vi "20150905 gyro+accel+ UL sensor+servo test.vi"() -> ()   [LabVIEW 2013]
uses:
  <vilib>/MakerHub/LINX/Public/Sensors/Accelerometer/MPU60X0/DeviceAddresses.ctl
  <vilib>/Analysis/baseanly.llb/Mean (DBL).vi
  <vilib>/MakerHub/LINX/Public/Sensors/Motion/Servo/Servo Open N Channels.vi
  <vilib>/MakerHub/LINX/Public/Sensors/Motion/Servo/Servo Close N Channels.vi
  <vilib>/MakerHub/LINX/Public/Sensors/Motion/Servo/Servo Set Pulse Width N Channels.vi
  <vilib>/addons/Time Series Analysis/Series Preprocess.llb/TSA Moving Average (Array).vi
  <vilib>/MakerHub/LINX/LMH-LINX.lvlib
  <vilib>/MakerHub/LINX/Public/Sensors/Motion/Servo/Servo.lvlib
  <vilib>/MakerHub/LINX/Public/Sensors/Ultrasonic/Ultrasonic.lvlib
  <vilib>/MakerHub/LINX/Public/Sensors/Accelerometer/MPU60X0/MPU60X0.lvlib
  <vilib>/addons/_Advanced Signal Processing/NI_AdvSigProcTSA.lvlib
  <vilib>/Analysis/NI_AALBase.lvlib
panel:
  in  "Moving avg?":bool
  out "Error Out":errorcluster
  out "Waveform Chart":cluster{"mean":dbl, "mean":dbl, "mean":dbl}(graph)
  out "mean 3":dbl format="%0.2f"
  out "mean 2":dbl format="%0.2f"
  out "mean":dbl format="%0.2f"
  out "x/y":T1
  in  "Servo Channels":u8[](array[numeric])=[2, 3, 4, 5, 6, 7, 8, 9, 10, 11, 12, 13]
  in  "error in (no error)":errorcluster
  out "Initialize OK?":bool=TRUE
  in  "Stop Button":bool
  in  "Pulse Widths (uS)":u16[](array[numeric])=[1400, 1400, 1300, 1600, 1500, 1400, 1500, 1500, 1400, 1400, 1200, 1500] min=600 max=2400 step=100
  in  "Serial Port":refnum<visa-resource-name>="COM10"
  # "up: CK"
  # "up: CK"
  # "up: CCK"
  # "up: CK"
  # "up: CK"
  # "up: CCK"
  # "up: CK"
  # "up: CK"
  # "up: CCK"
  # "up: CK"
  # "up: CK"
  # "up: CCK"
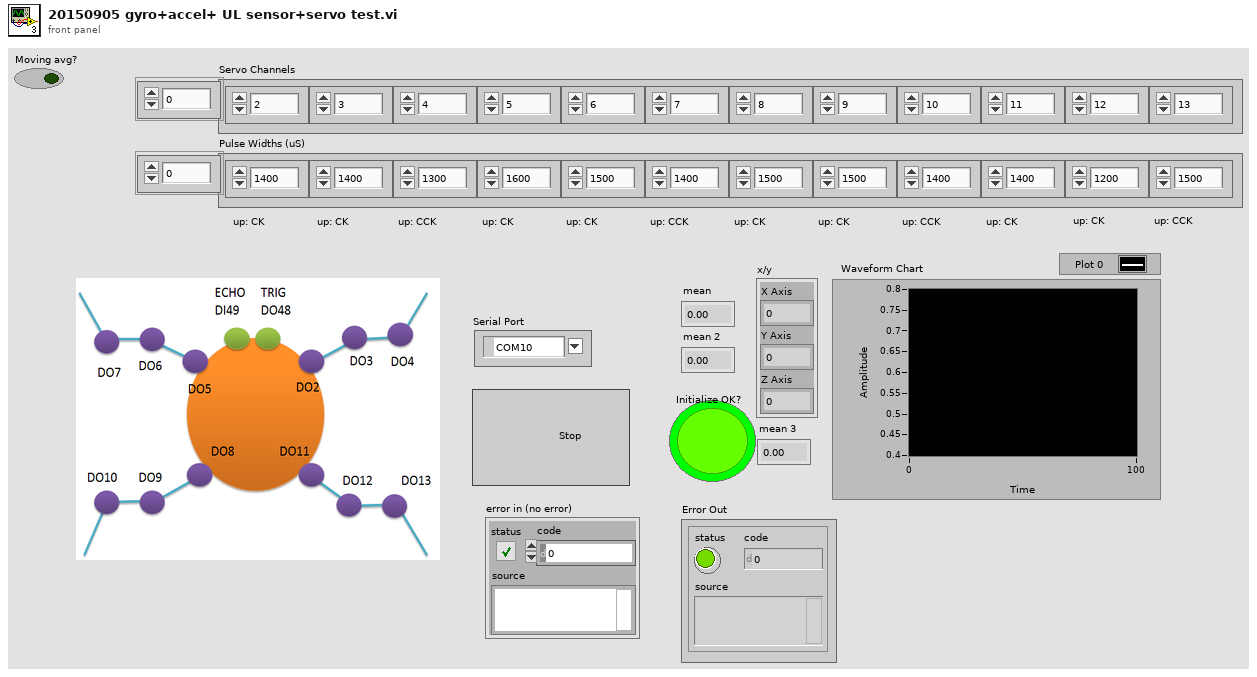
[diagram p1: front panel]
types:
  T1 = cluster{"X Axis":dbl, "Y Axis":dbl, "Z Axis":dbl}
  T2 = typedef "LMH-LINX.lvlib/MPU60X0.lvlib/DeviceAddresses.ctl" = enum16{"0x68", "0x69"}
  T3 = typedef "LMH-LINX.lvlib/LINX Ref.ctl" = cluster{"Platform":T4, "Interface":T5, "LINX Device Config":T6}
  T4 = typedef "LMH-LINX.lvlib/Platform.ctl" = enum16{"LINX", "myRIO"}
  T5 = typedef "LMH-LINX.lvlib/Interface.ctl" = enum16{"Serial", "TCP"}
  T6 = typedef "LMH-LINX.lvlib/Device.lvlib/LINX Device Config.ctl" = cluster{"Interface":T5, "COM Port":refnum<visa-resource-name>, "TCP Configuration":T7, "Device Family":u8, "Device ID":u8, "Device Name":string, "TCP Ref":refnum<k5>, "Channels":T8}
  T7 = typedef "LMH-LINX.lvlib/Device.lvlib/TCP Config.ctl" = cluster{"IP Address":string, "Port":u16}
  T8 = typedef "LMH-LINX.lvlib/Channels.ctl" = cluster{"DI":u8[], "DO":u8[], "AI":u8[], "AO":u8[], "PWM":u8[], "QE":u8[], "UART":u8[], "I2C 2":u8[], "SPI":u8[], "CAN":u8[], "Servo":u8[], "AI Ref (V)":dbl, "AO Ref (V)":dbl, "AO Resolution (Bits)":u8}
  T9 = cluster{"X Axis":i16, "Y Axis":i16, "Z Axis":i16}
  T10 = cluster{"X Axis":i32, "Y Axis":i32, "Z Axis":i32}
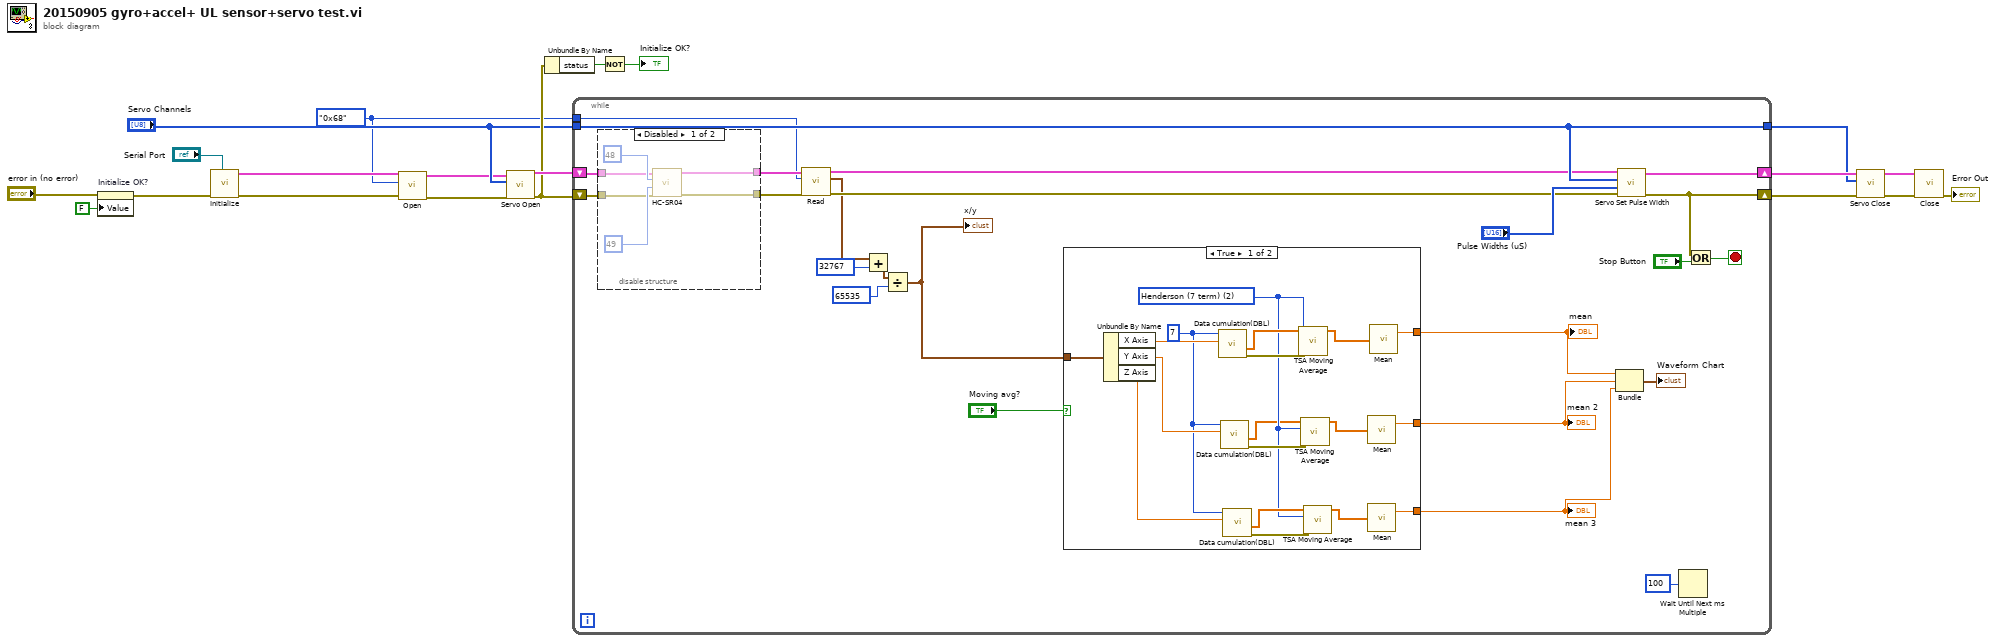
[diagram p0: block diagram]
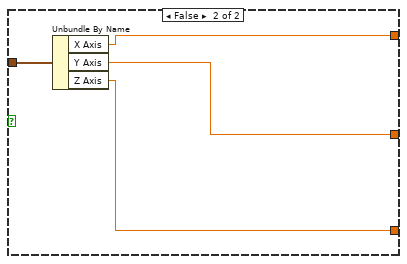
[diagram p2: hidden frame]
diagram:
  w2 = DeviceAddresses."0x68" ("Device Address")
  n1 = property on="Initialize OK?" class="Bool (strict)"(error in="error in (no error)", "Value"=FALSE ("Initialize OK?")) -> (error out=w11:errorcluster)  [unwired: 1 in, 1 out]
  n2 = call <vilib>:"Initialize.vi"("Serial Port"="Serial Port", "Error In"=w11) -> ("Error Out"=w5:errorcluster, "LINX Ref"=w6:T3)  [unwired: 7 in, 1 out]
  n3 = call <vilib>:"Open.vi"("Error In"=w5, "Device Address"=w2, "LINX Resource"=w6) -> ("Error Out"=w3:errorcluster, "LINX Resource"=w4:T3)  [unwired: 7 in]
  n4 = call-poly <vilib>:"Servo Open.vi"("Error In"=w3, "Servo Channels"="Servo Channels", "LINX Resource"=w4) -> ("Error Out"=w14:errorcluster, "LINX Resource"=w19:T3)  [unwired: 7 in]
  n5 = Unbundle By Name(w14) -> ("status"=w13:bool)
  n6 = while {
    shift-right: [w42] -> w15
    shift-left: w14 -> [w37]
    tunnel: "Servo Channels" -> [w40]
    shift-right: [w41] -> w18
    shift-left: w19 -> [w38]
    tunnel: [w40] -> w7
    tunnel: w2 -> [w31]
    stop <- w44 stop-if-true
    n7 = disable-structure shown="Disabled" {
      disable-tunnel: w38 -> [w70 w74]
      disable-tunnel: w37 -> [w69 w73]
      disable-tunnel: [w68 w73] -> w35
      disable-tunnel: [w67 w74] -> w33
      frame Disabled {
        n8 = call <vilib>:"HC-SR04.vi"("Error In"=w69, "Echo Pin (DI)"=u8 49, "Trig"=u8 48, "LINX Resource"=w70) -> ("Error Out"=w68:errorcluster, "LINX Resource"=w67:T3)  [unwired: 4 in, 2 out]
      }
      frame Enabled {
      }
    }
    n9 = call <vilib>:"Read.vi"("Error In"=w35, "Device Address"=w31, "LINX Resource"=w33) -> ("Error Out"=w34:errorcluster, "Acceleration Data"=w27:T9, "LINX Resource"=w32:T3)  [unwired: 4 in, 2 out]
    n10 = Add(x=w27, y=32767) -> (x+y=w30:T10)
    n11 = Divide(x=w30, y=65535) -> (x/y=w25:T1)
    "x/y" <- w25
    n12 = case shown="True" "Moving avg?" {
      tunnel: w25 -> [w62 w66]
      tunnel: [w47 w65] -> w24
      tunnel: [w46 w64] -> w23
      tunnel: [w45 w63] -> w22
      frame True {
        w52 = 2 items=["Spencer (15 term)"=1, "Henderson (7 term)"=2, "Henderson (9 term)"=3, "Henderson (13 term)"=4, "Henderson (23 term)"=5] ("method")
        w53 = 7 ("Sample length")
        n13 = Unbundle By Name(w62) -> ("X Axis"=w61:dbl, "Y Axis"=w55:dbl, "Z Axis"=w54:dbl)
        n14 = call "Data cumulation(DBL).vi"("Data in"=w61, "Sample length"=w53) -> ("error out"=w59:errorcluster, "Data out"=w60:dbl[])  [unwired: 6 in, 2 out]
        n15 = call "Data cumulation(DBL).vi"("Data in"=w55, "Sample length"=w53) -> ("error out"=w58:errorcluster, "Data out"=w51:dbl[])  [unwired: 6 in, 2 out]
        n16 = call "Data cumulation(DBL).vi"("Data in"=w54, "Sample length"=w53) -> ("error out"=w56:errorcluster, "Data out"=w57:dbl[])  [unwired: 6 in, 2 out]
        n17 = call-poly <vilib>:"TSA Moving Average.vi"("error in (no error)"=w59, "method"=w52, "Xt"=w60) -> ("Xt out"=w50:dbl[])  [unwired: 7 in, 1 out]
        n18 = call-poly <vilib>:"TSA Moving Average.vi"("error in (no error)"=w58, "method"=w52, "Xt"=w51) -> ("Xt out"=w49:dbl[])  [unwired: 7 in, 1 out]
        n19 = call-poly <vilib>:"TSA Moving Average.vi"("error in (no error)"=w56, "method"=w52, "Xt"=w57) -> ("Xt out"=w48:dbl[])  [unwired: 7 in, 1 out]
        n20 = call-poly <vilib>:"Mean.vi"("X"=w49) -> ("mean"=w46:dbl)  [unwired: 1 out]
        n21 = call-poly <vilib>:"Mean.vi"("X"=w48) -> ("mean"=w45:dbl)  [unwired: 1 out]
        n22 = call-poly <vilib>:"Mean.vi"("X"=w50) -> ("mean"=w47:dbl)  [unwired: 1 out]
      }
      frame False {
        n23 = Unbundle By Name(w66) -> ("X Axis"=w65:dbl, "Y Axis"=w64:dbl, "Z Axis"=w63:dbl)
      }
    }
    "mean" <- w24
    "mean 2" <- w23
    "mean 3" <- w22
    n24 = Bundle("X Axis"=w24, "Y Axis"=w23, "Z Axis"=w22) -> (→"Waveform Chart":T1)  [unwired: 1 in]
    n25 = call-poly <vilib>:"Servo Set Pulse Width.vi"("Error In"=w34, "Pulse Widths (uS)"="Pulse Widths (uS)", "Servo Channels"=w40, "LINX Resource"=w32) -> ("Error Out"=w42:errorcluster, "LINX Resource"=w41:T3)  [unwired: 6 in]
    n26 = Wait Until Next ms Multiple(millisecond multiple=u32 100) -> ()  [unwired: 1 out]
    n27 = Or(x=w42, y="Stop Button") -> (x .or. y?=w44:bool)
  }
  n28 = Not(x=w13) -> (.not. x?=→"Initialize OK?":bool)
  n29 = call-poly <vilib>:"Servo Close.vi"("Error In"=w15, "Servo Channels"=w7, "LINX Resource"=w18) -> ("Error Out"=w16:errorcluster, "LINX Resource"=w17:T3)  [unwired: 7 in]
  n30 = call <vilib>:"Close.vi"("Error In"=w16, "LINX Resource"=w17) -> ("Error Out"=→"Error Out":errorcluster)  [unwired: 8 in, 1 out]
